vi "Send gRPC to Main.vi"(8 "error in (no error)":errorcluster, 11 "CIFTemplatePlugin in":refnum<class "TemplatePlugin.lvclass">) -> (0 "error out":errorcluster, 3 "CIFTemplatePlugin out":refnum<class "TemplatePlugin.lvclass">)   [LabVIEW 2021, in "TemplatePlugin.lvclass"]
uses:
  TemplatePlugin.lvclass
  CIF-LVCore/src/CIFCore/Class/CIFCorePlugin.lvclass/CIFCorePlugin.ctl
  TemplatePlugin.lvclass/TemplatePlugin.ctl
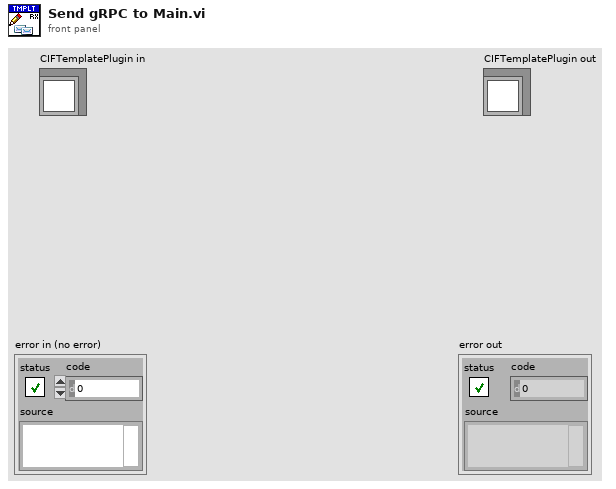
[diagram p1: front panel]
types:
  T1 = typedef "TemplatePlugin.lvclass/gRPC to Main Cyclic Data.ctl" = cluster{"Cyclic Data 1":i32}
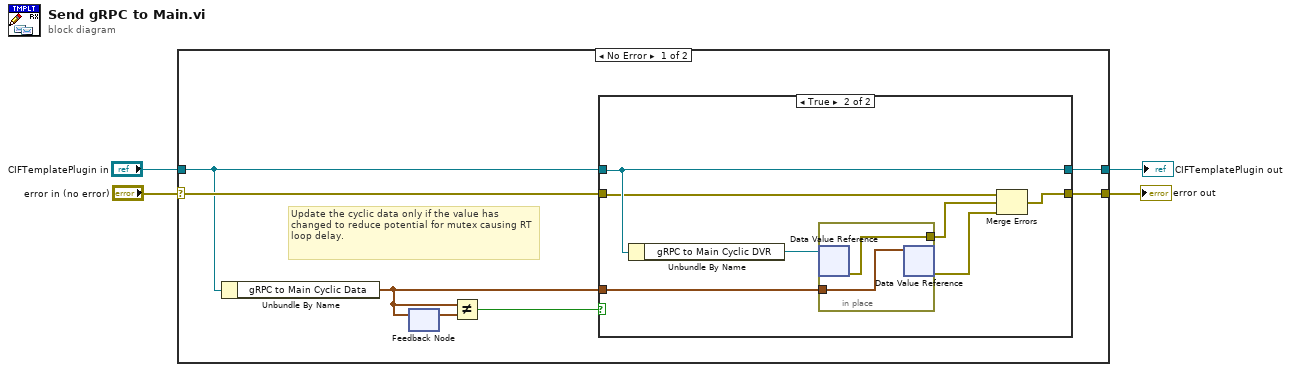
[diagram p0: block diagram]
diagram:
  n1 = case shown="No Error" "error in (no error)" {
    selector: "error in (no error)" -> [w7 w24]
    tunnel: [w8 w24] -> w3
    tunnel: [w9 w23] -> w1
    tunnel: "CIFTemplatePlugin in" -> [w6 w23]
    frame No Error {
      # "Update the cyclic data only if the value has changed to reduce potential for mutex causing RT loop delay."
      n2 = Unbundle By Name(w6) -> ("gRPC to Main Cyclic Data"=w10:T1)
      n3 = feedback-in #1(w10) -> ()
      n4 = feedback #1() -> (w11:T1)  [unwired: 1 in]
      n5 = Not Equal?(x=w10, y=w11) -> (x != y?=w5:bool)
      n6 = case shown="True" w5 {
        tunnel: w7 -> [w12 w17]
        tunnel: w6 -> [w13 w18]
        tunnel: w10 -> [_ w20]
        tunnel: [w13 w18] -> w9
        tunnel: [w12 w14] -> w8
        frame False {
        }
        frame True {
          n7 = Unbundle By Name(w18) -> ("gRPC to Main Cyclic DVR"=w19:refnum<data-value>)
          n8 = in-place {
            in-place-border: w20 -> [w22]
            in-place-border: [w21] -> w15
            n9 = in-place-dvr #2(w19) -> (w21:errorcluster)  [unwired: 1 out]
            n10 = in-place-dvr #2(w22) -> (w16:errorcluster)  [unwired: 1 out]
          }
          n11 = Merge Errors(w17, w15, w16) -> (w14:errorcluster)
        }
      }
    }
    frame Error {
    }
  }
  "error out" <- w3
  "CIFTemplatePlugin out" <- w1
